vi "BusInOut_write.vi"(8 "error in (no error)":errorcluster, 10 "value":dbl, 11 "BusInOut in":refnum<class "BusInOut.lvclass">) -> (0 "error out":errorcluster, 3 "BusInOut out":refnum<class "BusInOut.lvclass">)   [LabVIEW 2011, in "mbed_LVLibrary.lvlib" / "BusInOut.lvclass"]
uses:
  BusInOut.lvclass
  BusInOut.lvclass/BusInOut.ctl
  Transport Mechanisms/mbed/mbed.lvclass
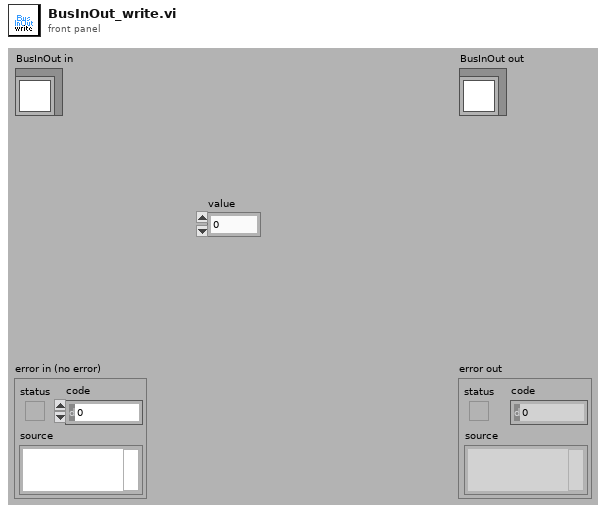
[diagram p1: front panel]
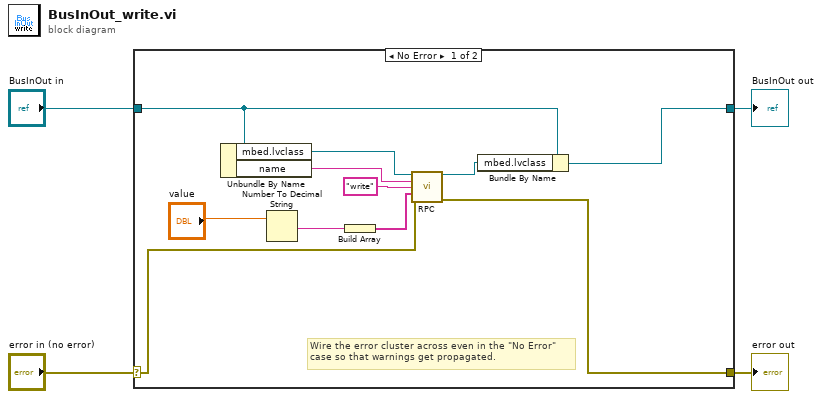
[diagram p0: block diagram]
diagram:
  n1 = case shown="No Error" "error in (no error)" {
    selector: "error in (no error)" -> [w6 w17]
    tunnel: [w5 w17] -> w3
    tunnel: [w8 w16] -> w1
    tunnel: "BusInOut in" -> [w9 w16]
    frame No Error {
      # "Wire the error cluster across even in the \"No Error\"\ncase so that warnings get propagated."
      n2 = Unbundle By Name(w9) -> ("mbed.lvclass"=w11:refnum<class "mbed.lvclass">, "name"=w10:string)
      n3 = Number To Decimal String(number="value") -> (decimal integer string=w14:string)  [unwired: 1 in]
      n4 = Build Array(w14) -> (w13:string[])
      n5 = call-dynamic "RPC.vi"("mbed in"=w11, "Name"=w10, "method"="write", "Args"=w13, "error in (no error)"=w6) -> ("mbed out"=w7:refnum<class "mbed.lvclass">, "error out"=w5:errorcluster)  [unwired: 8 in, 1 out]
      n6 = Bundle By Name(cluster=w9, "mbed.lvclass"=w7) -> (w8:refnum<class "BusInOut.lvclass">)
    }
    frame Error {
    }
  }
  "error out" <- w3
  "BusInOut out" <- w1
